vi "Read.vi"(8 "error in (no error)":errorcluster, 11 "Start Seq Command Config in":refnum<class "Start Seq Command Config.lvclass">) -> (0 "error out":errorcluster, 2 "Sequence":string, 3 "Start Seq Command Config out":refnum<class "Start Seq Command Config.lvclass">)   [LabVIEW 2020, in "VolatusSeqConfig.lvlib" / "Start Seq Command Config.lvclass"]
uses:
  Start Seq Command Config.lvclass
  Start Seq Command Config.lvclass/Start Seq Command Config.ctl
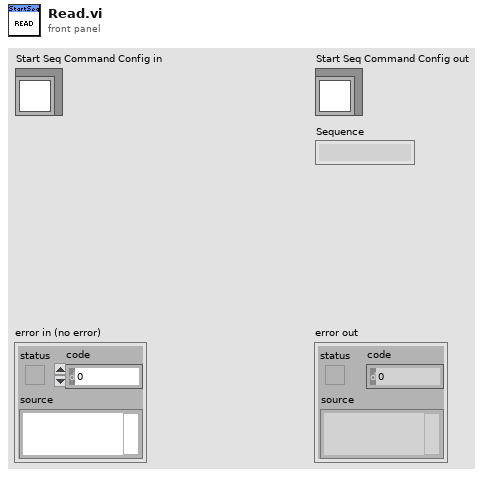
[diagram p1: front panel]
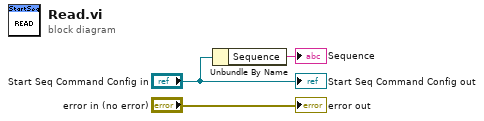
[diagram p0: block diagram]
diagram:
  n1 = Unbundle By Name("Start Seq Command Config in") -> ("Sequence"=→"Sequence":string)
  "error out" <- "error in (no error)"
  "Start Seq Command Config out" <- "Start Seq Command Config in"
